vi "user32_FlashWindow.vi"(7 "bInvert(F)":bool, 8 "错误输入（无错误）":errorcluster, 11 "hWnd":u32) -> (0 "错误输出":errorcluster, 2 "success?":bool, 3 "dup hWnd":u32)   [LabVIEW 2011]
doc: "闪烁显示指定窗口。这意味着窗口的标题和说明文字会发生变化，似乎从活动切换到非活动状态、或反向切换。通常对不活动的窗口应用这个函数，引起用户的注意。"
uses:
  user32.dll
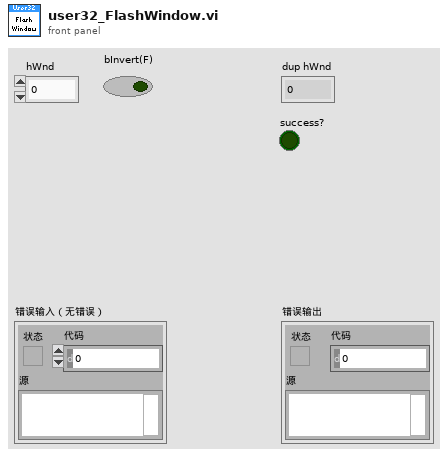
[diagram p1: front panel]
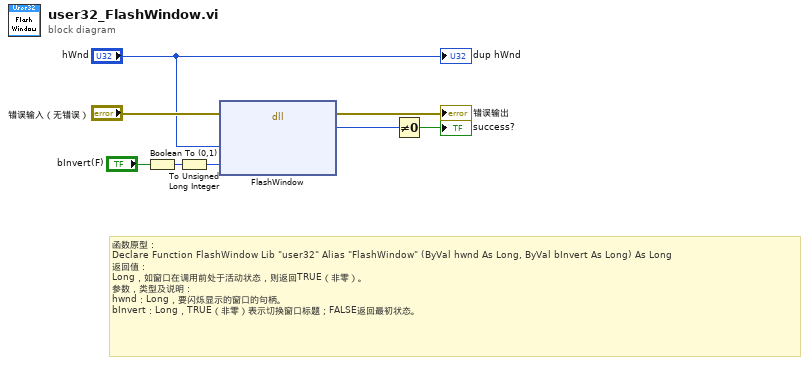
[diagram p0: block diagram]
diagram:
  # "函数原型：\nDeclare Function FlashWindow Lib \"user32\" Alias \"FlashWindow\" (ByVal hwnd As Long, ByVal bInvert As Long) As Long\n返回值：\nLong，如窗口在调用前处于活动状态，则返回TRUE（非零）。\n参数，类型及说明：\nhwnd：Long，要闪烁显示的窗口的句柄。\nbInvert：Long，TRUE（非零）表示切换窗口标题；FALSE返回最初状态。"
  n1 = Boolean To (0,1)(Boolean="bInvert(F)") -> (0, 1=w2:i16)
  n2 = To Unsigned Long Integer(number=w2) -> (unsigned 32bit integer=w1:u32)
  n3 = dll-call lib="user32.dll" fn="FlashWindow"(error in="错误输入（无错误）", "hWnd"="hWnd", "bInvert"=w1) -> (error out=→"错误输出":errorcluster, "Long"=w5:u32)  [unwired: 4 in, 1 out]
  n4 = Not Equal To 0?(x=w5) -> (x != 0?=→"success?":bool)
  "dup hWnd" <- "hWnd"
